vi "nanocal -- nuclear schottky fit V4.vi"() -> ()   [LabVIEW 2020] (continued)
0.149623565609 ,     0.141877858801 } , \r{    0.018836490895 ,     0.149623565609 ,     0.115522422306 } , \r{    0.022387211386 ,     0.149623565609 ,     0.093179863408 } , \r{    0.026607250598 ,     0.149623565609 ,     0.074729843493 } , \r{    0.031622776602 ,     0.149623565609 ,     0.059995877610 } , \r{    0.037583740429 ,     0.149623565609 ,     0.048775938318 } , \r{    0.044668359215 ,     0.149623565609 ,     0.040874020839 } , \r{    0.053088444423 ,     0.149623565609 ,     0.036127045463 } , \r{    0.063095734448 ,     0.149623565609 ,     0.034421884157 } , \r{    0.074989420933 ,     0.149623565609 ,     0.035699674200 } , \r{    0.089125093813 ,     0.149623565609 ,     0.039947569357 } , \r{    0.105925372518 ,     0.149623565609 ,     0.047180252600 } , \r{    0.125892541179 ,     0.149623565609 ,     0.057414385167 } , \r{    0.149623565609 ,     0.149623565609 ,     0.070639278795 } , \r{    0.177827941004 ,     0.149623565609 ,     0.086787357406 } , \r{    0.211348903984 ,     0.149623565609 ,     0.105708646760 } , \r{    0.251188643151 ,     0.149623565609 ,     0.127153912456 } , \r{    0.298538261892 ,     0.149623565609 ,     0.150770299518 } , \r{    0.354813389234 ,     0.149623565609 ,     0.176111225707 } , \r{    0.421696503429 ,     0.149623565609 ,     0.202659475022 } , \r{    0.501187233627 ,     0.149623565609 ,     0.229859851640 } , \r{    0.595662143529 ,     0.149623565609 ,     0.257156086913 } , \r{    0.707945784384 ,     0.149623565609 ,     0.284026281992 } , \r{    0.841395141645 ,     0.149623565609 ,     0.310012042831 } , \r{    0.001000000000 ,     0.177827941004 ,     0.740836835011 } , \r{    0.001188502227 ,     0.177827941004 ,     0.710329495354 } , \r{    0.001412537545 ,     0.177827941004 ,     0.677050447028 } , \r{    0.001678804018 ,     0.177827941004 ,     0.641106189632 } , \r{    0.001995262315 ,     0.177827941004 ,     0.602678568915 } , \r{    0.002371373706 ,     0.177827941004 ,     0.562039454503 } , \r{    0.002818382931 ,     0.177827941004 ,     0.519566808327 } , \r{    0.003349654392 ,     0.177827941004 ,     0.475755530109 } , \r{    0.003981071706 ,     0.177827941004 ,     0.431214355020 } , \r{    0.004731512590 ,     0.177827941004 ,     0.386642000254 } , \r{    0.005623413252 ,     0.177827941004 ,     0.342782601520 } , \r{    0.006683439176 ,     0.177827941004 ,     0.300369479723 } , \r{    0.007943282347 ,     0.177827941004 ,     0.260071698430 } , \r{    0.009440608763 ,     0.177827941004 ,     0.222455656817 } , \r{    0.011220184543 ,     0.177827941004 ,     0.187965930155 } , \r{    0.013335214322 ,     0.177827941004 ,     0.156921789373 } , \r{    0.015848931925 ,     0.177827941004 ,     0.129522861582 } , \r{    0.018836490895 ,     0.177827941004 ,     0.105859097961 } , \r{    0.022387211386 ,     0.177827941004 ,     0.085923590392 } , \r{    0.026607250598 ,     0.177827941004 ,     0.069629182896 } , \r{    0.031622776602 ,     0.177827941004 ,     0.056830202835 } , \r{    0.037583740429 ,     0.177827941004 ,     0.047349108968 } , \r{    0.044668359215 ,     0.177827941004 ,     0.041005320854 } , \r{    0.053088444423 ,     0.177827941004 ,     0.037641414898 } , \r{    0.063095734448 ,     0.177827941004 ,     0.037141549042 } , \r{    0.074989420933 ,     0.177827941004 ,     0.039438657457 } , \r{    0.089125093813 ,     0.177827941004 ,     0.044509677824 } , \r{    0.105925372518 ,     0.177827941004 ,     0.052360451062 } , \r{    0.125892541179 ,     0.177827941004 ,     0.063003162991 } , \r{    0.149623565609 ,     0.177827941004 ,     0.076429499384 } , \r{    0.177827941004 ,     0.177827941004 ,     0.092582860491 } , \r{    0.211348903984 ,     0.177827941004 ,     0.111333482638 } , \r{    0.251188643151 ,     0.177827941004 ,     0.132460756805 } , \r{    0.298538261892 ,     0.177827941004 ,     0.155646612919 } , \r{    0.354813389234 ,     0.177827941004 ,     0.180482156819 } , \r{    0.421696503429 ,     0.177827941004 ,     0.206487187930 } , \r{    0.501187233627 ,     0.177827941004 ,     0.233139638088 } , \r{    0.595662143529 ,     0.177827941004 ,     0.259910134828 } , \r{    0.707945784384 ,     0.177827941004 ,     0.286296242008 } , \r{    0.841395141645 ,     0.177827941004 ,     0.311851541843 } , \r{    0.001000000000 ,     0.211348903984 ,     0.658706462723 } , \r{    0.001188502227 ,     0.211348903984 ,     0.632229697281 } , \r{    0.001412537545 ,     0.211348903984 ,     0.603327363418 } , \r{    0.001678804018 ,     0.211348903984 ,     0.572087346120 } , \r{    0.001995262315 ,     0.211348903984 ,     0.538656633281 } , \r{    0.002371373706 ,     0.211348903984 ,     0.503252529375 } , \r{    0.002818382931 ,     0.211348903984 ,     0.466177332768 } , \r{    0.003349654392 ,     0.211348903984 ,     0.427831696047 } , \r{    0.003981071706 ,     0.211348903984 ,     0.388719014145 } , \r{    0.004731512590 ,     0.211348903984 ,     0.349433142339 } , \r{    0.005623413252 ,     0.211348903984 ,     0.310626218644 } , \r{    0.006683439176 ,     0.211348903984 ,     0.272961381709 } , \r{    0.007943282347 ,     0.211348903984 ,     0.237062250981 } , \r{    0.009440608763 ,     0.211348903984 ,     0.203472092487 } , \r{    0.011220184543 ,     0.211348903984 ,     0.172629846218 } , \r{    0.013335214322 ,     0.211348903984 ,     0.144862225297 } , \r{    0.015848931925 ,     0.211348903984 ,     0.120386368340 } , \r{    0.018836490895 ,     0.211348903984 ,     0.099317684423 } , \r{    0.022387211386 ,     0.211348903984 ,     0.081680417039 } , \r{    0.026607250598 ,     0.211348903984 ,     0.067421184763 } , \r{    0.031622776602 ,     0.211348903984 ,     0.056426796441 } , \r{    0.037583740429 ,     0.211348903984 ,     0.048546798094 } , \r{    0.044668359215 ,     0.211348903984 ,     0.043619100040 } , \r{    0.053088444423 ,     0.211348903984 ,     0.041494839043 } , \r{    0.063095734448 ,     0.211348903984 ,     0.042057671458 } , \r{    0.074989420933 ,     0.211348903984 ,     0.045233607293 } , \r{    0.089125093813 ,     0.211348903984 ,     0.050989777453 } , \r{    0.105925372518 ,     0.211348903984 ,     0.059322962241 } , \r{    0.125892541179 ,     0.211348903984 ,     0.070240293599 } , \r{    0.149623565609 ,     0.211348903984 ,     0.083735123682 } , \r{    0.177827941004 ,     0.211348903984 ,     0.099761216436 } , \r{    0.211348903984 ,     0.211348903984 ,     0.118208753852 } , \r{    0.251188643151 ,     0.211348903984 ,     0.138886076738 } , \r{    0.298538261892 ,     0.211348903984 ,     0.161510944813 } , \r{    0.354813389234 ,     0.211348903984 ,     0.185713860663 } , \r{    0.421696503429 ,     0.211348903984 ,     0.211053773929 } , \r{    0.501187233627 ,     0.211348903984 ,     0.237043967586 } , \r{    0.595662143529 ,     0.211348903984 ,     0.263183941094 } , \r{    0.707945784384 ,     0.211348903984 ,     0.288992188714 } , \r{    0.841395141645 ,     0.211348903984 ,     0.314035081981 } , \r{    0.001000000000 ,     0.251188643151 ,     0.583753974070 } , \r{    0.001188502227 ,     0.251188643151 ,     0.561057464983 } , \r{    0.001412537545 ,     0.251188643151 ,     0.536261953482 } , \r{    0.001678804018 ,     0.251188643151 ,     0.509441674684 } , \r{    0.001995262315 ,     0.251188643151 ,     0.480716417964 } , \r{    0.002371373706 ,     0.251188643151 ,     0.450258891242 } , \r{    0.002818382931 ,     0.251188643151 ,     0.418306756758 } , \r{    0.003349654392 ,     0.251188643151 ,     0.385176391666 } , \r{    0.003981071706 ,     0.251188643151 ,     0.351272300628 } , \r{    0.004731512590 ,     0.251188643151 ,     0.317084637215 } , \r{    0.005623413252 ,     0.251188643151 ,     0.283169393408 } , \r{    0.006683439176 ,     0.251188643151 ,     0.250111957470 } , \r{    0.007943282347 ,     0.251188643151 ,     0.218482233638 } , \r{    0.009440608763 ,     0.251188643151 ,     0.188793416013 } , \r{    0.011220184543 ,     0.251188643151 ,     0.161473822961 } , \r{    0.013335214322 ,     0.251188643151 ,     0.136854159170 } , \r{    0.015848931925 ,     0.251188643151 ,     0.115166529542 } , \r{    0.018836490895 ,     0.251188643151 ,     0.096549850207 } , \r{    0.022387211386 ,     0.251188643151 ,     0.081058241465 } , \r{    0.026607250598 ,     0.251188643151 ,     0.068671793768 } , \r{    0.031622776602 ,     0.251188643151 ,     0.059310729766 } , \r{    0.037583740429 ,     0.251188643151 ,     0.052853849353 } , \r{    0.044668359215 ,     0.251188643151 ,     0.049160578455 } , \r{    0.053088444423 ,     0.251188643151 ,     0.048093842246 } , \r{    0.063095734448 ,     0.251188643151 ,     0.049539555202 } , \r{    0.074989420933 ,     0.251188643151 ,     0.053418665177 } , \r{    0.089125093813 ,     0.251188643151 ,     0.059689373296 } , \r{    0.105925372518 ,     0.251188643151 ,     0.068339460616 } , \r{    0.125892541179 ,     0.251188643151 ,     0.079370510719 } , \r{    0.149623565609 ,     0.251188643151 ,     0.092776735099 } , \r{    0.177827941004 ,     0.251188643151 ,     0.108521376077 } , \r{    0.211348903984 ,     0.251188643151 ,     0.126513873499 } , \r{    0.251188643151 ,     0.251188643151 ,     0.146591332212 } , \r{    0.298538261892 ,     0.251188643151 ,     0.168507891467 } , \r{    0.354813389234 ,     0.251188643151 ,     0.191934786010 } , \r{    0.421696503429 ,     0.251188643151 ,     0.216472066639 } , \r{    0.501187233627 ,     0.251188643151 ,     0.241670603037 } , \r{    0.595662143529 ,     0.251188643151 ,     0.267060904339 } , \r{    0.707945784384 ,     0.251188643151 ,     0.292184101542 } , \r{    0.841395141645 ,     0.251188643151 ,     0.316620409071 } , \r{    0.001000000000 ,     0.298538261892 ,     0.517704935038 } , \r{    0.001188502227 ,     0.298538261892 ,     0.498483642507 } , \r{    0.001412537545 ,     0.298538261892 ,     0.477463151719 } , \r{    0.001678804018 ,     0.298538261892 ,     0.454708039811 } , \r{    0.001995262315 ,     0.298538261892 ,     0.430317916888 } , \r{    0.002371373706 ,     0.298538261892 ,     0.404430957044 } , \r{    0.002818382931 ,     0.298538261892 ,     0.377232485595 } , \r{    0.003349654392 ,     0.298538261892 ,     0.348967315706 } , \r{    0.003981071706 ,     0.298538261892 ,     0.319951559176 } , \r{    0.004731512590 ,     0.298538261892 ,     0.290577377217 } , \r{    0.005623413252 ,     0.298538261892 ,     0.261304285049 } , \r{    0.006683439176 ,     0.298538261892 ,     0.232634443257 } , \r{    0.007943282347 ,     0.298538261892 ,     0.205075982287 } , \r{    0.009440608763 ,     0.298538261892 ,     0.179104073008 } , \r{    0.011220184543 ,     0.298538261892 ,     0.155130036145 } , \r{    0.013335214322 ,     0.298538261892 ,     0.133483847148 } , \r{    0.015848931925 ,     0.298538261892 ,     0.114408951404 } , \r{    0.018836490895 ,     0.298538261892 ,     0.098064811086 } , \r{    0.022387211386 ,     0.298538261892 ,     0.084533116759 } , \r{    0.026607250598 ,     0.298538261892 ,     0.073826084038 } , \r{    0.031622776602 ,     0.298538261892 ,     0.065897330233 } , \r{    0.037583740429 ,     0.298538261892 ,     0.060656379298 } , \r{    0.044668359215 ,     0.298538261892 ,     0.057986900287 } , \r{    0.053088444423 ,     0.298538261892 ,     0.057766973425 } , \r{    0.063095734448 ,     0.298538261892 ,     0.059887999585 } , \r{    0.074989420933 ,     0.298538261892 ,     0.064268325763 } , \r{    0.089125093813 ,     0.298538261892 ,     0.070858633213 } , \r{    0.105925372518 ,     0.298538261892 ,     0.079638111104 } , \r{    0.125892541179 ,     0.298538261892 ,     0.090602425808 } , \r{    0.149623565609 ,     0.298538261892 ,     0.103745757535 } , \r{    0.177827941004 ,     0.298538261892 ,     0.119039662023 } , \r{    0.211348903984 ,     0.298538261892 ,     0.136411689542 } , \r{    0.251188643151 ,     0.298538261892 ,     0.155726935779 } , \r{    0.298538261892 ,     0.298538261892 ,     0.176775860178 } , \r{    0.354813389234 ,     0.298538261892 ,     0.199271268192 } , \r{    0.421696503429 ,     0.298538261892 ,     0.222855986016 } , \r{    0.501187233627 ,     0.298538261892 ,     0.247120689274 } , \r{    0.595662143529 ,     0.298538261892 ,     0.271629244883 } , \r{    0.707945784384 ,     0.298538261892 ,     0.295947480550 } , \r{    0.841395141645 ,     0.298538261892 ,     0.319670904915 } , \r{    0.001000000000 ,     0.354813389234 ,     0.461802046903 } , \r{    0.001188502227 ,     0.354813389234 ,     0.445715861517 } , \r{    0.001412537545 ,     0.354813389234 ,     0.428098537544 } , \r{    0.001678804018 ,     0.354813389234 ,     0.409007654015 } , \r{    0.001995262315 ,     0.354813389234 ,     0.388528341511 } , \r{    0.002371373706 ,     0.354813389234 ,     0.366773369859 } , \r{    0.002818382931 ,     0.354813389234 ,     0.343887989903 } , \r{    0.003349654392 ,     0.354813389234 ,     0.320059548601 } , \r{    0.003981071706 ,     0.354813389234 ,     0.295529331319 } , \r{    0.004731512590 ,     0.354813389234 ,     0.270601601307 } , \r{    0.005623413252 ,     0.354813389234 ,     0.245643669355 } , \r{    0.006683439176 ,     0.354813389234 ,     0.221072447582 } , \r{    0.007943282347 ,     0.354813389234 ,     0.197327737812 } , \r{    0.009440608763 ,     0.354813389234 ,     0.174838486318 } , \r{    0.011220184543 ,     0.354813389234 ,     0.153991480792 } , \r{    0.013335214322 ,     0.354813389234 ,     0.135109942669 } , \r{    0.015848931925 ,     0.354813389234 ,     0.118443882956 } , \r{    0.018836490895 ,     0.354813389234 ,     0.104169302093 } , \r{    0.022387211386 ,     0.354813389234 ,     0.092392082586 } , \r{    0.026607250598 ,     0.354813389234 ,     0.083154079639 } , \r{    0.031622776602 ,     0.354813389234 ,     0.076441152816 } , \r{    0.037583740429 ,     0.354813389234 ,     0.072194056197 } , \r{    0.044668359215 ,     0.354813389234 ,     0.070322824798 } , \r{    0.053088444423 ,     0.354813389234 ,     0.070723930547 } , \r{    0.063095734448 ,     0.354813389234 ,     0.073297794987 } , \r{    0.074989420933 ,     0.354813389234 ,     0.077963185268 } , \r{    0.089125093813 ,     0.354813389234 ,     0.084665252670 } , \r{    0.105925372518 ,     0.354813389234 ,     0.093375422231 } , \r{    0.125892541179 ,     0.354813389234 ,     0.104083257620 } , \r{    0.149623565609 ,     0.354813389234 ,     0.116781962397 } , \r{    0.177827941004 ,     0.354813389234 ,     0.131449965768 } , \r{    0.211348903984 ,     0.354813389234 ,     0.148031298487 } , \r{    0.251188643151 ,     0.354813389234 ,     0.166417619532 } , \r{    0.298538261892 ,     0.354813389234 ,     0.186434918726 } , \r{    0.354813389234 ,     0.354813389234 ,     0.207837754480 } , \r{    0.421696503429 ,     0.354813389234 ,     0.230312971944 } , \r{    0.501187233627 ,     0.354813389234 ,     0.253493157225 } , \r{    0.595662143529 ,     0.354813389234 ,     0.276978084046 } , \r{    0.707945784384 ,     0.354813389234 ,     0.300360774991 } , \r{    0.841395141645 ,     0.354813389234 ,     0.323254041024 } , \r{    0.001000000000 ,     0.421696503429 ,     0.416711745146 } , \r{    0.001188502227 ,     0.421696503429 ,     0.403405424373 } , \r{    0.001412537545 ,     0.421696503429 ,     0.388801996550 } , \r{    0.001678804018 ,     0.421696503429 ,     0.372953265916 } , \r{    0.001995262315 ,     0.421696503429 ,     0.355933853019 } , \r{    0.002371373706 ,     0.421696503429 ,     0.337838521448 } , \r{    0.002818382931 ,     0.421696503429 ,     0.318783451795 } , \r{    0.003349654392 ,     0.421696503429 ,     0.298912458920 } , \r{    0.003981071706 ,     0.421696503429 ,     0.278407081902 } , \r{    0.004731512590 ,     0.421696503429 ,     0.257497137785 } , \r{    0.005623413252 ,     0.421696503429 ,     0.236466581026 } , \r{    0.006683439176 ,     0.421696503429 ,     0.215649499411 } , \r{    0.007943282347 ,     0.421696503429 ,     0.195413771552 } , \r{    0.009440608763 ,     0.421696503429 ,     0.176134888784 } , \r{    0.011220184543 ,     0.421696503429 ,     0.158167059297 } , \r{    0.013335214322 ,     0.421696503429 ,     0.141819622963 } , \r{    0.015848931925 ,     0.421696503429 ,     0.127343271395 } , \r{    0.018836490895 ,     0.421696503429 ,     0.114925528459 } , \r{    0.022387211386 ,     0.421696503429 ,     0.104692064238 } , \r{    0.026607250598 ,     0.421696503429 ,     0.096710743330 } , \r{    0.031622776602 ,     0.421696503429 ,     0.090997273470 } , \r{    0.037583740429 ,     0.421696503429 ,     0.087522948802 } , \r{    0.044668359215 ,     0.421696503429 ,     0.086225360489 } , \r{    0.053088444423 ,     0.421696503429 ,     0.087022135267 } , \r{    0.063095734448 ,     0.421696503429 ,     0.089826294113 } , \r{    0.074989420933 ,     0.421696503429 ,     0.094560484261 } , \r{    0.089125093813 ,     0.421696503429 ,     0.101166907408 } , \r{    0.105925372518 ,     0.421696503429 ,     0.109610554380 } , \r{    0.125892541179 ,     0.421696503429 ,     0.119874971535 } , \r{    0.149623565609 ,     0.421696503429 ,     0.131951445202 } , \r{    0.177827941004 ,     0.421696503429 ,     0.145823593529 } , \r{    0.211348903984 ,     0.421696503429 ,     0.161449818861 } , \r{    0.251188643151 ,     0.421696503429 ,     0.178746221763 } , \r{    0.298538261892 ,     0.421696503429 ,     0.197572693944 } , \r{    0.354813389234 ,     0.421696503429 ,     0.217724892271 } , \r{    0.421696503429 ,     0.421696503429 ,     0.238934275633 } , \r{    0.501187233627 ,     0.421696503429 ,     0.260877135971 } , \r{    0.595662143529 ,     0.421696503429 ,     0.283191791372 } , \r{    0.707945784384 ,     0.421696503429 ,     0.305501396843 } , \r{    0.841395141645 ,     0.421696503429 ,     0.327438742692 } , \r{    0.001000000000 ,     0.501187233627 ,     0.382498963678 } , \r{    0.001188502227 ,     0.501187233627 ,     0.371619717619 } , \r{    0.001412537545 ,     0.501187233627 ,     0.359643822955 } , \r{    0.001678804018 ,     0.501187233627 ,     0.346617257902 } , \r{    0.001995262315 ,     0.501187233627 ,     0.332606289949 } , \r{    0.002371373706 ,     0.501187233627 ,     0.317692910823 } , \r{    0.002818382931 ,     0.501187233627 ,     0.301973094158 } , \r{    0.003349654392 ,     0.501187233627 ,     0.285559516092 } , \r{    0.003981071706 ,     0.501187233627 ,     0.268588823278 } , \r{    0.004731512590 ,     0.501187233627 ,     0.251231514228 } , \r{    0.005623413252 ,     0.501187233627 ,     0.233700619039 } , \r{    0.006683439176 ,     0.501187233627 ,     0.216254420067 } , \r{    0.007943282347 ,     0.501187233627 ,     0.199189383598 } , \r{    0.009440608763 ,     0.501187233627 ,     0.182822738472 } , \r{    0.011220184543 ,     0.501187233627 ,     0.167468647881 } , \r{    0.013335214322 ,     0.501187233627 ,     0.153414887674 } , \r{    0.015848931925 ,     0.501187233627 ,     0.140906053700 } , \r{    0.018836490895 ,     0.501187233627 ,     0.130135312395 } , \r{    0.022387211386 ,     0.501187233627 ,     0.121242839483 } , \r{    0.026607250598 ,     0.501187233627 ,     0.114317848157 } , \r{    0.031622776602 ,     0.501187233627 ,     0.109402268895 } , \r{    0.037583740429 ,     0.501187233627 ,     0.106495908924 } , \r{    0.044668359215 ,     0.501187233627 ,     0.105563878676 } , \r{    0.053088444423 ,     0.501187233627 ,     0.106546864479 } , \r{    0.063095734448 ,     0.501187233627 ,     0.109373749657 } , \r{    0.074989420933 ,     0.501187233627 ,     0.113974731139 } , \r{    0.089125093813 ,     0.501187233627 ,     0.120292172945 } , \r{    0.105925372518 ,     0.501187233627 ,     0.128286535662 } , \r{    0.125892541179 ,     0.501187233627 ,     0.137935828301 } , \r{    0.149623565609 ,     0.501187233627 ,     0.149228595672 } , \r{    0.177827941004 ,     0.501187233627 ,     0.162151793987 } , \r{    0.211348903984 ,     0.501187233627 ,     0.176675657566 } , \r{    0.251188643151 ,     0.501187233627 ,     0.192737921294 } , \r{    0.298538261892 ,     0.501187233627 ,     0.210229847437 } , \r{    0.354813389234 ,     0.501187233627 ,     0.228986534293 } , \r{    0.421696503429 ,     0.501187233627 ,     0.248783743287 } , \r{    0.501187233627 ,     0.501187233627 ,     0.269342666886 } , \r{    0.595662143529 ,     0.501187233627 ,     0.290342647138 } , \r{    0.707945784384 ,     0.501187233627 ,     0.311440212229 } , \r{    0.841395141645 ,     0.501187233627 ,     0.332291480224 } , \r{    0.001000000000 ,     0.595662143529 ,     0.358671219729 } , \r{    0.001188502227 ,     0.595662143529 ,     0.349882157487 } , \r{    0.001412537545 ,     0.595662143529 ,     0.340166106960 } , \r{    0.001678804018 ,     0.595662143529 ,     0.329562278481 } , \r{    0.001995262315 ,     0.595662143529 ,     0.318129160990 } , \r{    0.002371373706 ,     0.595662143529 ,     0.305939009622 } , \r{    0.002818382931 ,     0.595662143529 ,     0.293073891561 } , \r{    0.003349654392 ,     0.595662143529 ,     0.279625268208 } , \r{    0.003981071706 ,     0.595662143529 ,     0.265698037639 } , \r{    0.004731512590 ,     0.595662143529 ,     0.251418323562 } , \r{    0.005623413252 ,     0.595662143529 ,     0.236942532027 } , \r{    0.006683439176 ,     0.595662143529 ,     0.222463874544 } , \r{    0.007943282347 ,     0.595662143529 ,     0.208212349848 } , \r{    0.009440608763 ,     0.595662143529 ,     0.194445756283 } , \r{    0.011220184543 ,     0.595662143529 ,     0.181432674722 } , \r{    0.013335214322 ,     0.595662143529 ,     0.169432005561 } , \r{    0.015848931925 ,     0.595662143529 ,     0.158675053766 } , \r{    0.018836490895 ,     0.595662143529 ,     0.149354151962 } , \r{    0.022387211386 ,     0.595662143529 ,     0.141618074195 } , \r{    0.026607250598 ,     0.595662143529 ,     0.135571936594 } , \r{    0.031622776602 ,     0.595662143529 ,     0.131279200532 } , \r{    0.037583740429 ,     0.595662143529 ,     0.128764831083 } , \r{    0.044668359215 ,     0.595662143529 ,     0.128020006149 } , \r{    0.053088444423 ,     0.595662143529 ,     0.129009158286 } , \r{    0.063095734448 ,     0.595662143529 ,     0.131679552968 } , \r{    0.074989420933 ,     0.595662143529 ,     0.135972465039 } , \r{    0.089125093813 ,     0.595662143529 ,     0.141833892977 } , \r{    0.105925372518 ,     0.595662143529 ,     0.149222265177 } , \r{    0.125892541179 ,     0.595662143529 ,     0.158111070502 } , \r{    0.149623565609 ,     0.595662143529 ,     0.168485578802 } , \r{    0.177827941004 ,     0.595662143529 ,     0.180334217329 } , \r{    0.211348903984 ,     0.595662143529 ,     0.193636197284 } , \r{    0.251188643151 ,     0.595662143529 ,     0.208347473588 } , \r{    0.298538261892 ,     0.595662143529 ,     0.224387257855 } , \r{    0.354813389234 ,     0.595662143529 ,     0.241627329089 } , \r{    0.421696503429 ,     0.595662143529 ,     0.259886293333 } , \r{    0.501187233627 ,     0.595662143529 ,     0.278930488434 } , \r{    0.595662143529 ,     0.595662143529 ,     0.298482226423 } , \r{    0.707945784384 ,     0.595662143529 ,     0.318234646419 } , \r{    0.841395141645 ,     0.595662143529 ,     0.337871047210 } , \r{    0.001000000000 ,     0.707945784384 ,     0.344279898358 } , \r{    0.001188502227 ,     0.707945784384 ,     0.337268699566 } , \r{    0.001412537545 ,     0.707945784384 ,     0.329473699264 } , \r{    0.001678804018 ,     0.707945784384 ,     0.320926024993 } , \r{    0.001995262315 ,     0.707945784384 ,     0.311675849778 } , \r{    0.002371373706 ,     0.707945784384 ,     0.301786837397 } , \r{    0.002818382931 ,     0.707945784384 ,     0.291330912344 } , \r{    0.003349654392 ,     0.707945784384 ,     0.280385385593 } , \r{    0.003981071706 ,     0.707945784384 ,     0.269033897700 } , \r{    0.004731512590 ,     0.707945784384 ,     0.257371418611 } , \r{    0.005623413252 ,     0.707945784384 ,     0.245512000288 } , \r{    0.006683439176 ,     0.707945784384 ,     0.233596579236 } , \r{    0.007943282347 ,     0.707945784384 ,     0.221797353004 } , \r{    0.009440608763 ,     0.707945784384 ,     0.210315629843 } , \r{    0.011220184543 ,     0.707945784384 ,     0.199371982981 } , \r{    0.013335214322 ,     0.707945784384 ,     0.189190656542 } , \r{    0.015848931925 ,     0.707945784384 ,     0.179982798322 } , \r{    0.018836490895 ,     0.707945784384 ,     0.171933260980 } , \r{    0.022387211386 ,     0.707945784384 ,     0.165193225134 } , \r{    0.026607250598 ,     0.707945784384 ,     0.159877837071 } , \r{    0.031622776602 ,     0.707945784384 ,     0.156066657041 } , \r{    0.037583740429 ,     0.707945784384 ,     0.153805323136 } , \r{    0.044668359215 ,     0.707945784384 ,     0.153108205787 } , \r{    0.053088444423 ,     0.707945784384 ,     0.153962709019 } , \r{    0.063095734448 ,     0.707945784384 ,     0.156335838322 } , \r{    0.074989420933 ,     0.707945784384 ,     0.160182884907 } , \r{    0.089125093813 ,     0.707945784384 ,     0.165456998590 } , \r{    0.105925372518 ,     0.707945784384 ,     0.172117574384 } , \r{    0.125892541179 ,     0.707945784384 ,     0.180135244398 } , \r{    0.149623565609 ,     0.707945784384 ,     0.189491979043 } , \r{    0.177827941004 ,     0.707945784384 ,     0.200176026648 } , \r{    0.211348903984 ,     0.707945784384 ,     0.212172607819 } , \r{    0.251188643151 ,     0.707945784384 ,     0.225452043162 } , \r{    0.298538261892 ,     0.707945784384 ,     0.239957297520 } , \r{    0.354813389234 ,     0.707945784384 ,     0.255592977770 } , \r{    0.421696503429 ,     0.707945784384 ,     0.272217779186 } , \r{    0.501187233627 ,     0.707945784384 ,     0.289642152560 } , \r{    0.595662143529 ,     0.707945784384 ,     0.307632344406 } , \r{    0.707945784384 ,     0.707945784384 ,     0.325920877303 } , \r{    0.841395141645 ,     0.707945784384 ,     0.344222221305 } , \r{    0.001000000000 ,     0.841395141645 ,     0.338057235803 } , \r{    0.001188502227 ,     0.841395141645 ,     0.332540491283 } , \r{    0.001412537545 ,     0.841395141645 ,     0.326361600129 } , \r{    0.001678804018 ,     0.841395141645 ,     0.319542452651 } , \r{    0.001995262315 ,     0.841395141645 ,     0.312123858442 } , \r{    0.002371373706 ,     0.841395141645 ,     0.304160702070 } , \r{    0.002818382931 ,     0.841395141645 ,     0.295716376983 } , \r{    0.003349654392 ,     0.841395141645 ,     0.286858333364 } , \r{    0.003981071706 ,     0.841395141645 ,     0.277656438145 } , \r{    0.004731512590 ,     0.841395141645 ,     0.268185069466 } , \r{    0.005623413252 ,     0.841395141645 ,     0.258528621406 } , \r{    0.006683439176 ,     0.841395141645 ,     0.248788759073 } , \r{    0.007943282347 ,     0.841395141645 ,     0.239090758823 } , \r{    0.009440608763 ,     0.841395141645 ,     0.229585965790 } , \r{    0.011220184543 ,     0.841395141645 ,     0.220448175740 } , \r{    0.013335214322 ,     0.841395141645 ,     0.211863777840 } , \r{    0.015848931925 ,     0.841395141645 ,     0.204018144929 } , \r{    0.018836490895 ,     0.841395141645 ,     0.197082412434 } , \r{    0.022387211386 ,     0.841395141645 ,     0.191204095814 } , \r{    0.026607250598 ,     0.841395141645 ,     0.186502488296 } , \r{    0.031622776602 ,     0.841395141645 ,     0.183067526296 } , \r{    0.037583740429 ,     0.841395141645 ,     0.180960295139 } , \r{    0.044668359215 ,     0.841395141645 ,     0.180214276074 } , \r{    0.053088444423 ,     0.841395141645 ,     0.180837571382 } , \r{    0.063095734448 ,     0.841395141645 ,     0.182816821978 } , \r{    0.074989420933 ,     0.841395141645 ,     0.186123219061 } , \r{    0.089125093813 ,     0.841395141645 ,     0.190720178045 } , \r{    0.105925372518 ,     0.841395141645 ,     0.196571299937 } , \r{    0.125892541179 ,     0.841395141645 ,     0.203646663557 } , \r{    0.149623565609 ,     0.841395141645 ,     0.211925622011 } , \r{    0.177827941004 ,     0.841395141645 ,     0.221395103699 } , \r{    0.211348903984 ,     0.841395141645 ,     0.232043555101 } , \r{    0.251188643151 ,     0.841395141645 ,     0.243851634664 } , \r{    0.298538261892 ,     0.841395141645 ,     0.256781317268 } , \r{    0.354813389234 ,     0.841395141645 ,     0.270765245362 } , \r{    0.421696503429 ,     0.841395141645 ,     0.285698155030 } , \r{    0.501187233627 ,     0.841395141645 ,     0.301432093581 } , \r{    0.595662143529 ,     0.841395141645 ,     0.317776809420 } , \r{    0.707945784384 ,     0.841395141645 ,     0.334505973391 } , \r{    0.841395141645 ,     0.841395141645 ,     0.351368812895 } , \r }   "
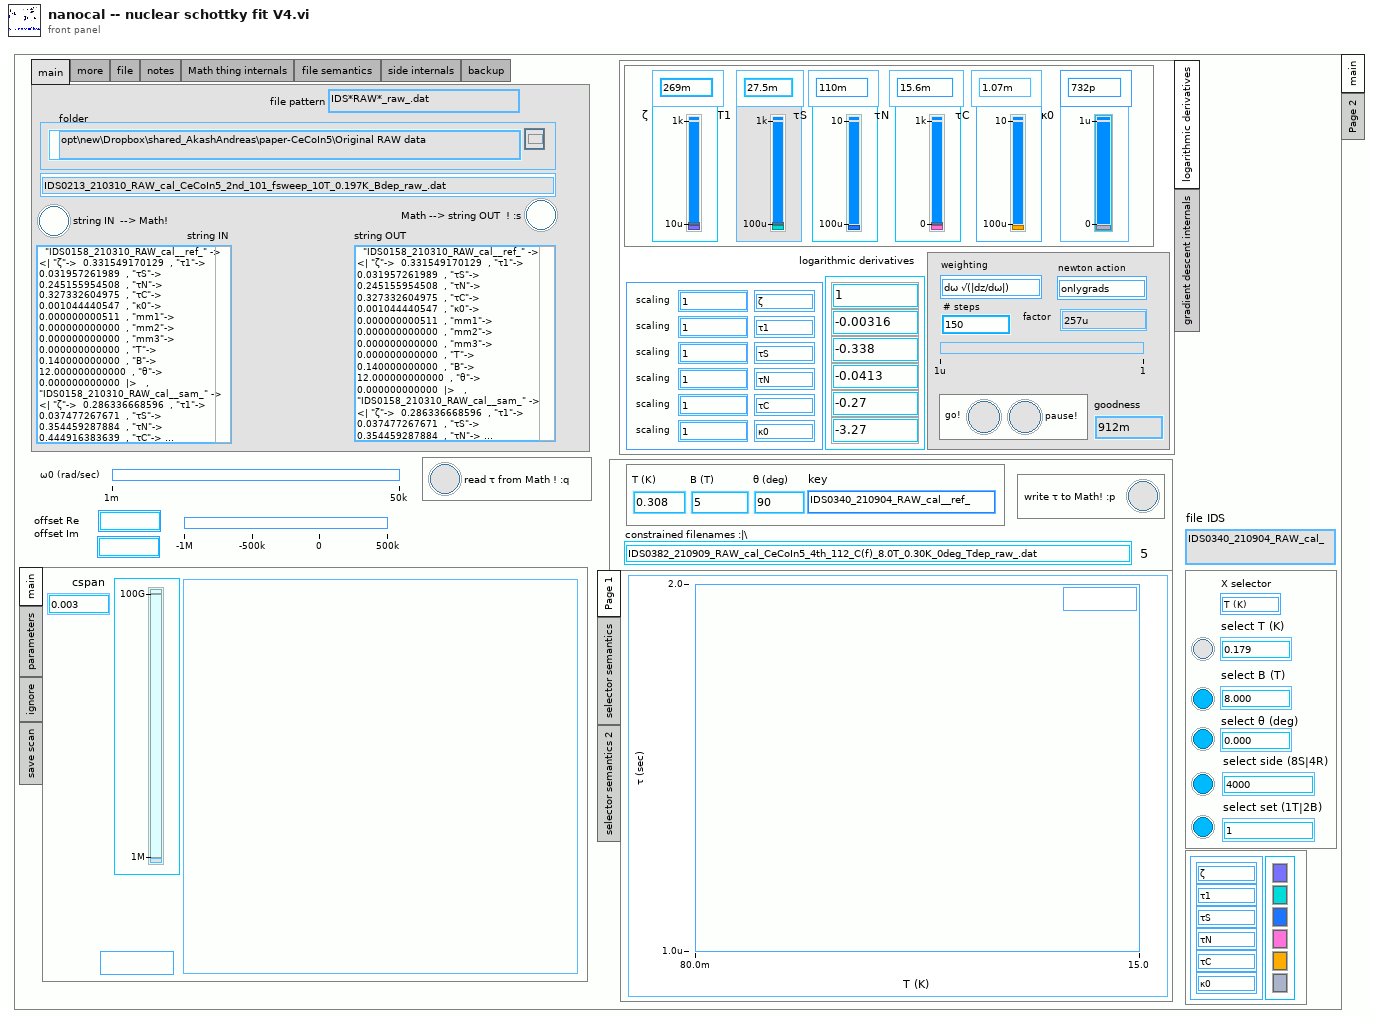
[diagram p1: front panel]
types:
  T1 = enum32{"main", "parameters", "ignore", "save scan"}
  T2 = typedef "cursor winow.ctl" = cluster{"left":dbl, "right ":dbl, "center":dbl, "window":dbl, "cursors":i32[], "relative":i32, "absolute":i32, "fixed vertical offset":dbl, "vertical offset":dbl, "skew":dbl, "default window frac":dbl, "kind":enum16{"symmetric", "skewed", "fancy"}, "skew.left":dbl, "skew.right":dbl, "Plot ref":refnum<vi>, "wing order":enum16{"forw", "back"}}
  T3 = typedef "show-win- control.ctl" = cluster{"cen (Hz)":dbl, "win (Hz)":dbl, "left (Hz)":dbl, "right (Hz)":dbl}
  T4 = typedef "NI_Gmath.lvlib/stopping criteria.ctl" = cluster{"function tolerance":dbl, "parameter tolerance":dbl, "max iterations":i32, "max function calls":i32, "gradient tolerance":dbl, "max time (sec)":dbl}
  T5 = typedef "3-lorentzian-parameters.ctl" = enum16{"ζ", "τ1", "τS", "τN", "τC", "κ0", "m1", "m2", "m3", "T (K)", "B (T)", "θ (deg)", "side (S|R)", "change (B|T)"}
  T6 = typedef "filename-pattern.ctl" = cluster{"prefix":string, "group":string}
  T7 = enum32{"logarithmic derivatives", "gradient descent internals"}
  T8 = typedef "nanocal-goodness-weighting-strategy.ctl" = enum16{"dω", "dω √(|dz/dω|)", "dω |dz/dω|", "phase", "andreas", "sum"}
  T9 = typedef "3-lorentzian-heat-response action.ctl" = enum16{"calc R", "create string", "calc m1m2m3", "dζ", "dT1", "dτS", "dτN", "dτC", "d-all", "dκ0", "T(K)", "m1", "m2", "m3", "parse string", "θ (deg)", "B (T)", "onlygrads", "newton", "create emty string"}
  T10 = enum32{"Page 1", "selector semantics", "selector semantics 2"}
  T11 = typedef "nameformattingitem.ctl" = enum16{"name", "nameL", "units", "prec"}
  T12 = enum32{"main", "more", "file", "notes", "Math thing internals", "file semantics ", "side internals", "backup"}
  T13 = typedef "nanocal_data_read_format.ctl" = enum16{"as is", "add - ω", "full rydh", "raw nanocal"}
  T14 = typedef "nanocal_side_selector.ctl" = enum16{"sam", "ref"}
  T15 = typedef "filename-action.ctl" = enum16{"rewrite", "parse", "force pattern", "uniquenum", "get T", "get B", "get ind", "get deg", "get name", "get folder", "get extension", "get basename", "get side", "get change", "getID", "getIDStock"}
  T16 = typedef "cursor action.ctl" = enum16{"range", "read", "write", "check", "zoom out", "smart zoom out", "zoom to aspect ratio 1", "zoom to win", "zoom out 20%", "zoom in 20%", "-empty", "smart zoom out&aspect", "move range left 20%", "move range right 20%", "move range up 20%", "move range down 20%", "zoom to X win", "zoom to Y win", "zoom out X", "zoom out Y", "zoom in X", "zoom in Y", "check plot scale", "set plot color", "set Xlabel", "set Ylabel", "set cursor color"}
  T17 = typedef "cursor window action.ctl" = enum16{"balance", "h. offset change", "cursor moves", "change center", "change window", "init", "check", "reset", "set y to middle", "idle", "-write all Y", "-write left.X", "-write center.X", "-write right.X", "-write all X", "-change center", "-change window", "-change skew", "-read cursor 2", "-read cursor 1", "-read cursor 0", "-read all cursors", "-reset", "-read plot scale", "-set y to middle", "-Q: center.Y is visible", "-Q: window is visible", "-parse center.Y", "-right left from center", "-left move", "-right move", "-set center.Y", "-empty", "-set cursors to default", "-check", "-write center.Y", "-copy cursor 1", "-copy cursor 0", "-copy cursor 2", "move right", "move left", "shrink", "broaden", "skew up", "skew down", "-write plot scale", "zoom X", "change cen&win", "zoom to all data", "color--red", "color--green", "color--yellow", "read", "zoom out", "zoom in", "slide right", "slide left", "set range aspect ratio to 1"}
  T18 = typedef "mathematica string map action.ctl" = enum16{"create string", "calc m1m2m3", "parse string"}
  T19 = typedef "publisher action.ctl" = enum16{"set", "get", "init", "check"}
  T20 = typedef "cursor sate.ctl" = enum16{"normal", "alert", "fuzzy", "interesting", "boring", "colored"}
  T21 = typedef "3-lorentzian-parameters -- action.ctl" = enum16{"to array", "to parameters"}
  T22 = typedef "NI_Gmath.lvlib/objective function data.ctl" = variant
  T23 = typedef "LVMapReplaceAction.ctl" = enum32{"Modify Entry only if found", "Add or Modify Entry", "Delete Entry"}
  T24 = typedef "file -- read-write control.ctl" = enum16{"read", "write all", "append one line"}
  T25 = typedef "array -- freq-voltage transformations action.ctl" = enum16{"as is", "add -ω", "sort ω", "2 x ω", "R-phase(deg) to Re-Im", "select ω>0", "labview file str"}
  T26 = typedef "nanocal_raw_file_manage_action_V1.ctl" = enum16{"read S side", "read R side", "read meta", "read_names"}
  T27 = typedef "KM_file -- read-write control.ctl" = enum16{"read", "write all", "append one line"}
  T28 = typedef "array action.ctl" = enum16{"generate range", "generate log range"}
  T29 = typedef "LVRangeTypeDef.ctl" = cluster{"Minimum":dbl, "Maximum":dbl, "Increment":dbl, "Minor Increment":dbl, "Start":dbl}
  T30 = typedef "2Dwindow.ctl" = cluster{"window y":dbl, "center x":dbl, "center y":dbl, "window x":dbl}
  T31 = typedef "eventvkey.ctl" = enum16{"ASCII", "Enter", "Return", "Shift", "Ctrl", "Alt", "Cmd", "Opt", "Caps", "NumLock", "Clear", "Break", "Up", "Down", "Left", "Right", "Insert", "Delete", "Home", "End", "PageUp", "PageDown", "Escape", "Help", "Pause", "ScrollLock", "F1", "F2", "F3", "F4", "F5", "F6", "F7", "F8", "F9", "F10", "F11", "F12", "F13", "F14", "F15", "F16", "F17", "F18", "F19", "F20", "F21", "F22", "F23", "F24", "Play", "VolumeUp", "VolumeDown", "Mute", "Two Byte Char"}
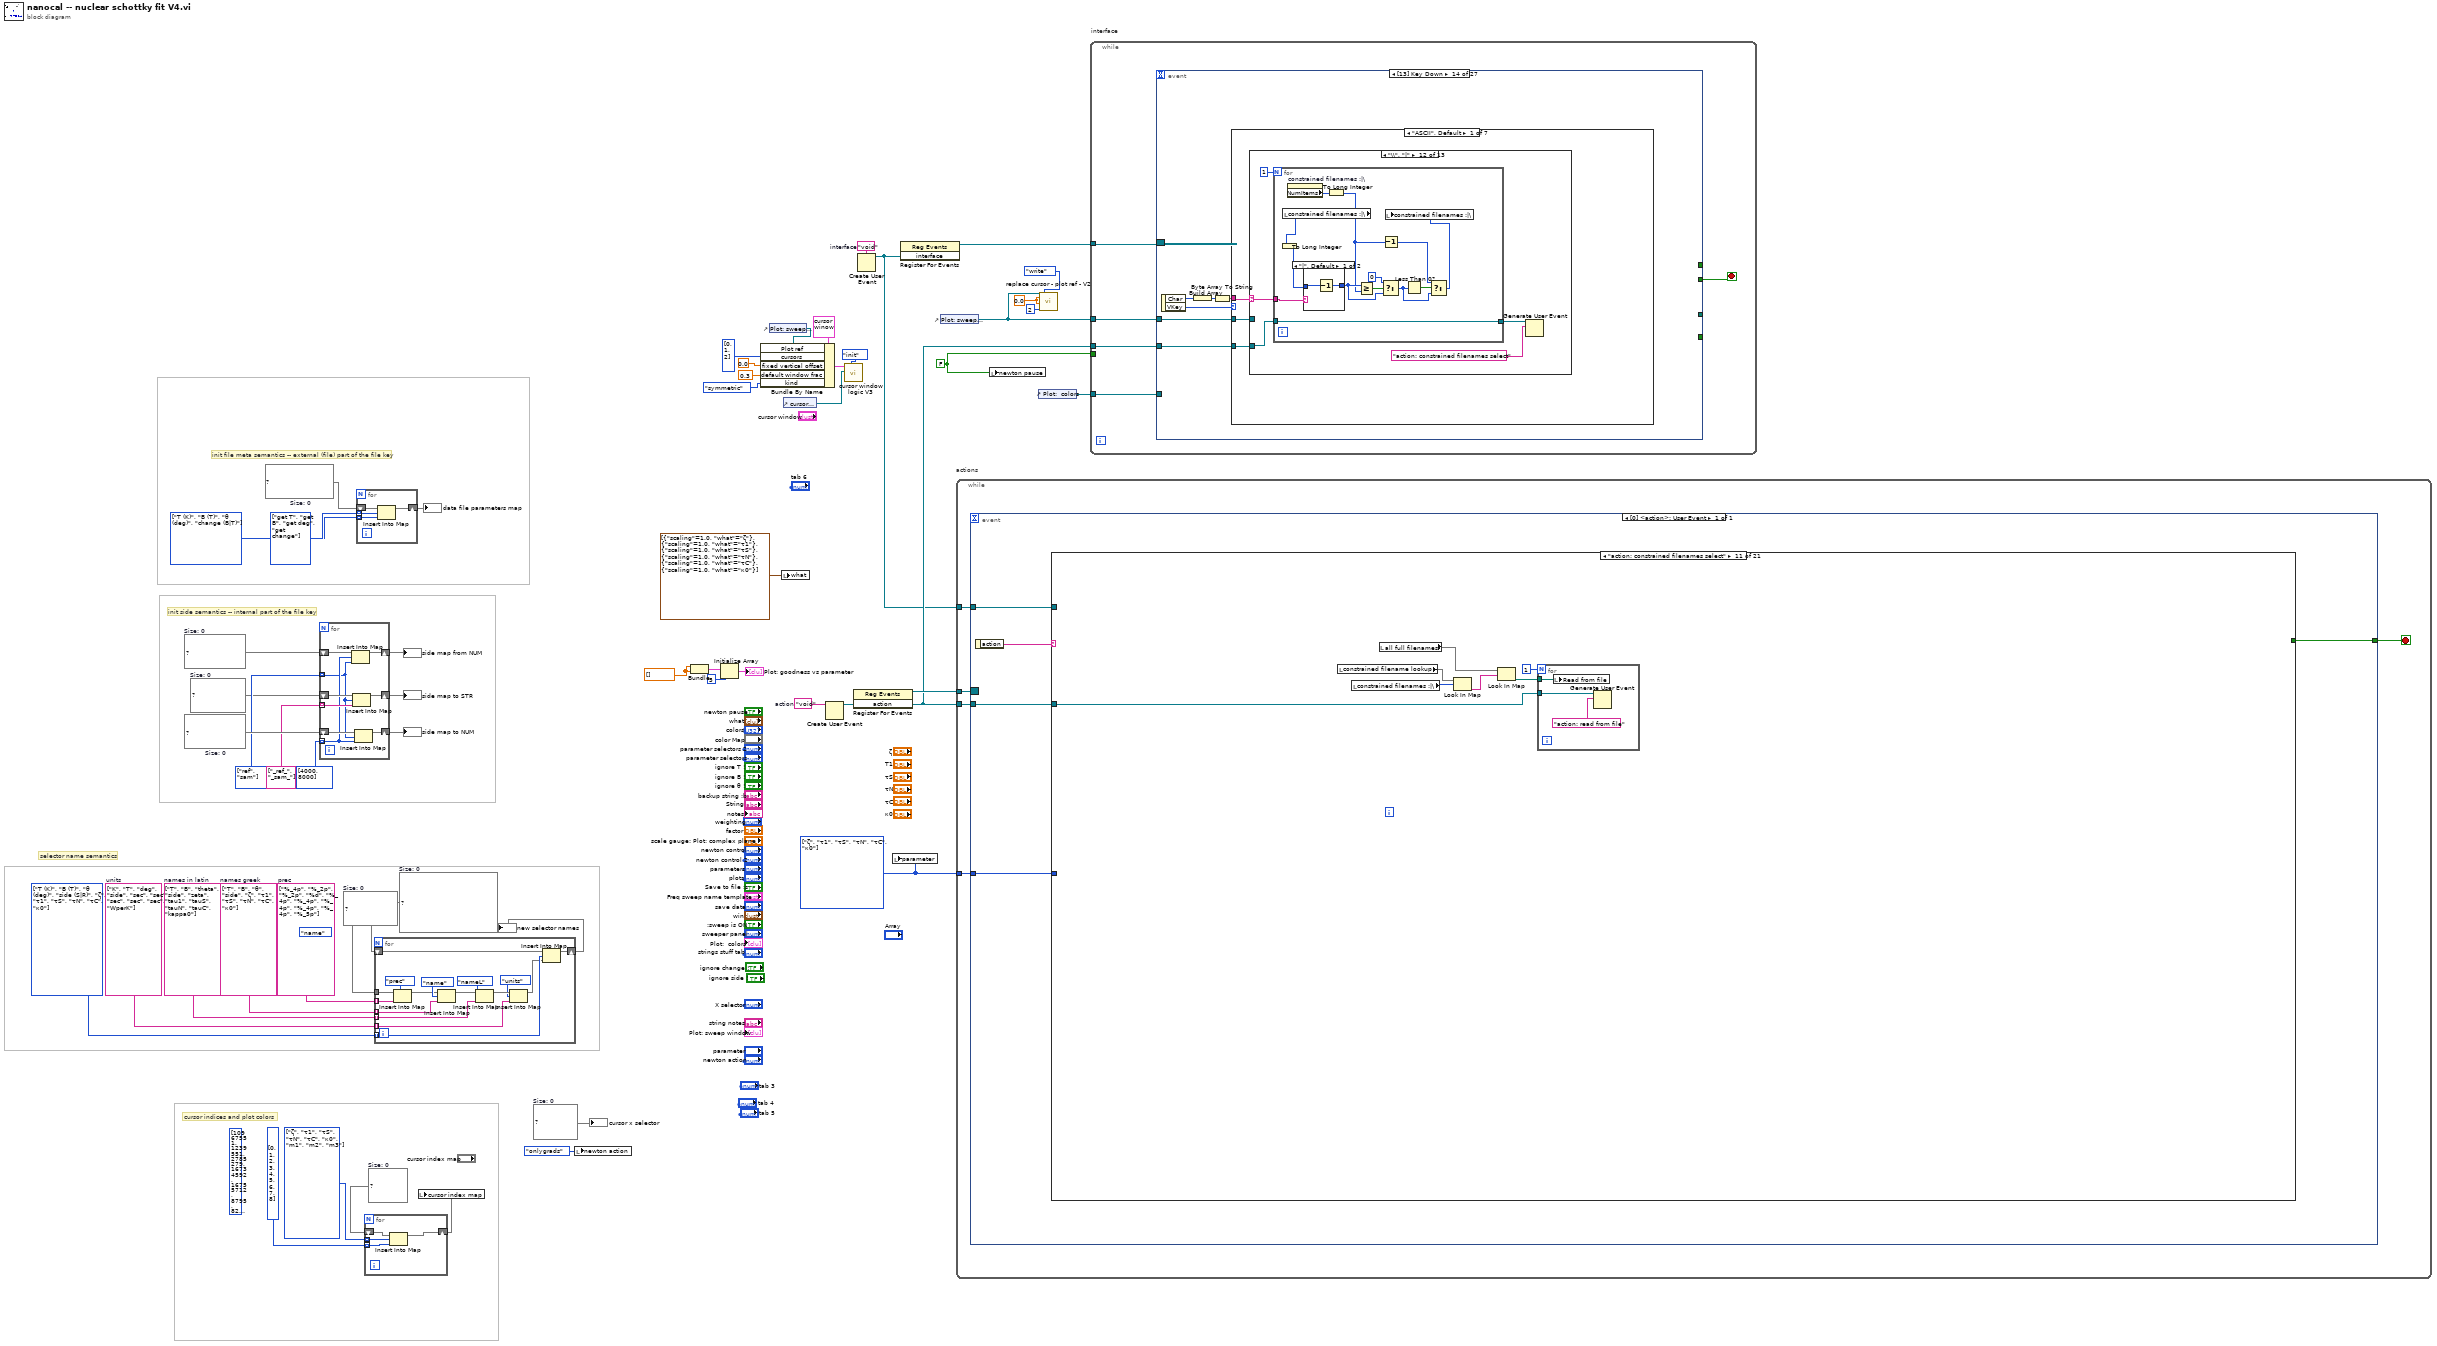
[diagram p0: block diagram]
diagram:
  w1 = T15[] [enum."get T", enum."get B", enum."get deg", enum."get change"] items=["rewrite", "parse", "force pattern", "uniquenum", "get T", "get B", "get ind", "get deg", "get name", "get folder", "get extension", "get basename", "get side", "get change", "getID", "getIDStock"]
  w3 = map{T5, T15} {}  # Size: 0
  w2 = T5[] [enum."T (K)", enum."B (T)", enum."θ (deg)", enum."change (B|T)"] items=["ζ", "τ1", "τS", "τN", "τC", "κ0", "m1", "m2", "m3", "T (K)", "B (T)", "θ (deg)", "side (S|R)", "change (B|T)"]
  w6 = map{i32, T14} {}  # Size: 0
  w8 = map{T14, string} {}  # Size: 0
  w9 = T14[] [enum."ref", enum."sam"] items=["sam", "ref"]
  w13 = map{T14, i32} {}  # Size: 0
  w14 = string[] ["%_4p", "%_2p", "%_2p", "%d", "%_4p", "%_4p", "%_4p", "%_4p", "%_4p", "%_5p"]  # prec
  w18 = map{T11, string} {}  # Size: 0
  (unwired) nameformattingitem."name" ("name formatting item")
  w16 = string[] ["K", "T", "deg", "side", "sec", "sec", "sec", "sec", "sec", "WperK"]  # units
